vi "Send_Ack_Nack.vi"(8 "Postition to Be Set in":i32[](array[numeric]), 9 "VISA resource name":refnum<visa-resource-name>) -> (2 "Output":enum16{"Error", "NACK", "ACK", "First Send"}(ring), 3 "VISA Out":refnum<visa-resource-name>)   [LabVIEW 2017]
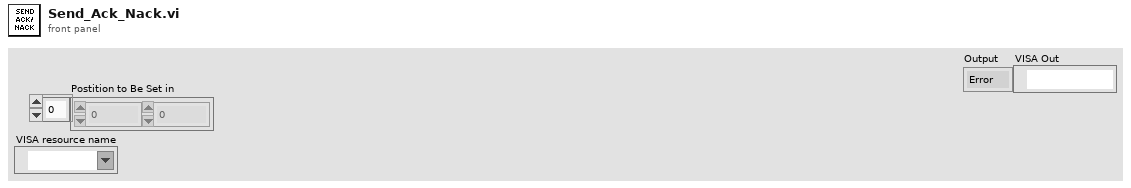
[diagram p1: front panel]
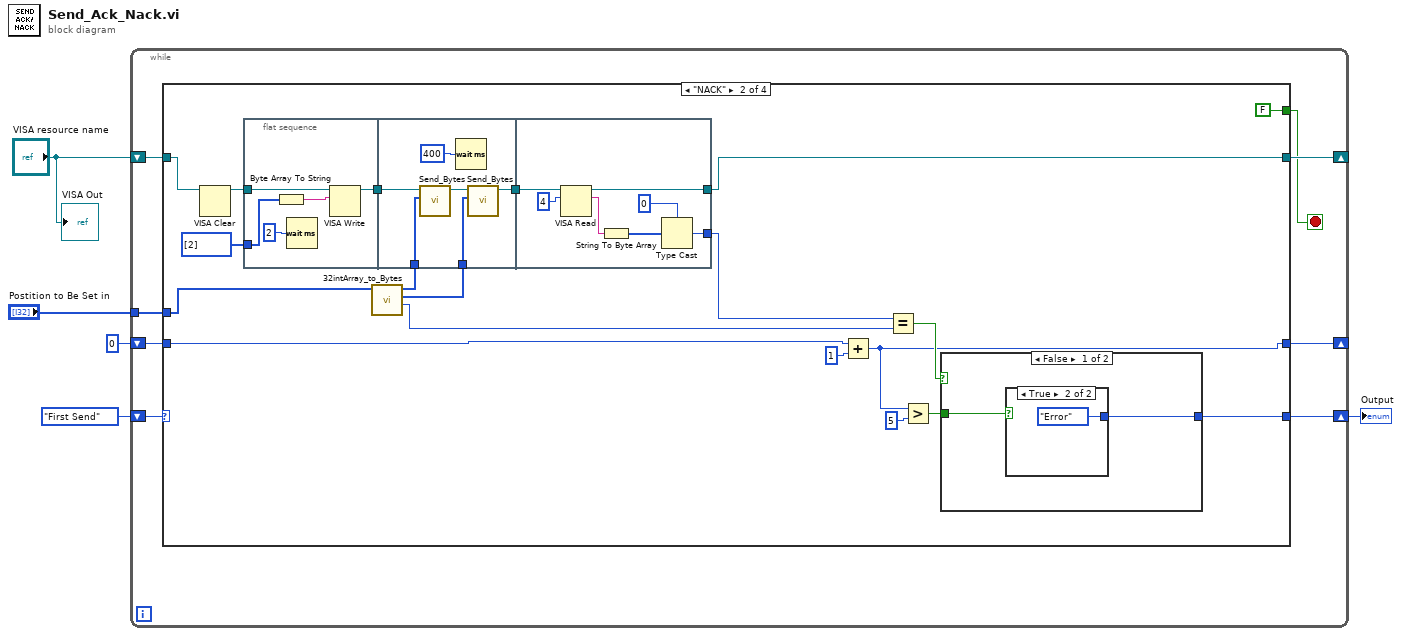
[diagram p0: block diagram]
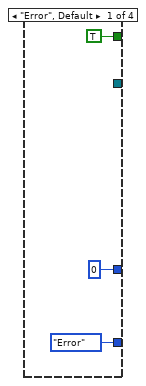
[diagram p2: hidden frame]
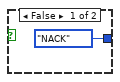
[diagram p3: hidden frame]
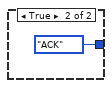
[diagram p4: hidden frame]
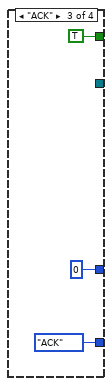
[diagram p5: hidden frame]
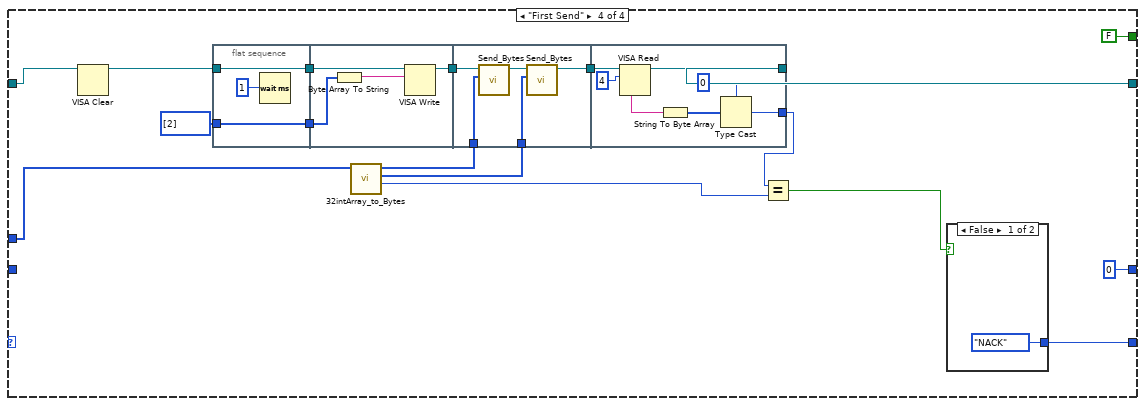
[diagram p6: hidden frame]
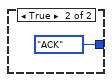
[diagram p7: hidden frame]
diagram:
  n1 = while {
    shift-right: [w9] -> w1
    shift-left: enum16{"Error", "NACK", "ACK", "First Send"}."First Send" -> [w13]
    tunnel: "Postition to Be Set in" -> [w12]
    shift-right: [w6] -> _
    shift-left: 0 -> [w7]
    shift-right: [w11] -> _
    shift-left: "VISA resource name" -> [w10]
    stop <- w8 stop-if-true
    n2 = case shown="\"NACK\"" w13 {
      tunnel: w12 -> [_ w25 _ w73]
      tunnel: [_ w24 _ w70] -> w11
      tunnel: w10 -> [_ w26 _ w63]
      tunnel: [enum16{"Error", "NACK", "ACK", "First Send"}."Error" w23 enum16{"Error", "NACK", "ACK", "First Send"}."ACK" w68] -> w9
      tunnel: [TRUE FALSE TRUE FALSE] -> w8
      tunnel: w7 -> [_ w22 _ _]
      tunnel: [0 w18 0 0] -> w6
      frame "Error", Default {
      }
      frame "NACK" {
        n3 = VISA Clear(VISA resource name=w26) -> (VISA resource name out=w27:refnum<visa-resource-name>)  [unwired: 1 in, 1 out]
        n4 = flat-sequence {
          tunnel: [w45] -> w35
          tunnel: w27 -> [w44]
          tunnel: u8[] [2] -> [w43]
          tunnel: w35 -> [w46]
          tunnel: w29 -> [w48]
          tunnel: [w49] -> w34
          tunnel: w28 -> [w51]
          tunnel: [w57] -> w24
          tunnel: w34 -> [w58]
          tunnel: [w52] -> w32
          frame #0 {
            n5 = Byte Array To String(unsigned byte array=w43) -> (string=w42:string)
            n6 = Wait (ms)(milliseconds to wait=u32 2) -> ()  [unwired: 1 out]
            n7 = VISA Write(VISA resource name=w44, write buffer=w42) -> (VISA resource name out=w45:refnum<visa-resource-name>)  [unwired: 1 in, 2 out]
          }
          frame #1 {
            n8 = call "Send_Bytes.vi"("Array1"=w51, "VISA resource name"=w46) -> ("VISA resource"=w50:refnum<visa-resource-name>)  [unwired: 9 in]
            n9 = Wait (ms)(milliseconds to wait=u32 400) -> ()  [unwired: 1 out]
            n10 = call "Send_Bytes.vi"("Array1"=w48, "VISA resource name"=w50) -> ("VISA resource"=w49:refnum<visa-resource-name>)  [unwired: 9 in]
          }
          frame #2 {
            n11 = VISA Read(VISA resource name=w58, byte count=u32 4) -> (VISA resource name out=w57:refnum<visa-resource-name>, read buffer=w56:string)  [unwired: 1 in, 2 out]
            n12 = String To Byte Array(string=w56) -> (unsigned byte array=w55:u8[])
            n13 = Type Cast(type=0, x=w55) -> (*(type *) &x=w52:i32)
          }
        }
        n14 = call "32intArray_to_Bytes.vi"("Postition to Be Set"=w25) -> ("result"=w31:i32, "Array2"=w29:u8[], "Array1"=w28:u8[])  [unwired: 8 in]
        n15 = Add(x=w22, y=1) -> (x+y=w18:i32)
        n16 = Equal?(x=w32, y=w31) -> (x = y?=w33:bool)
        n17 = Greater?(x=w18, y=5) -> (0:w19:bool)
        n18 = case shown="False" w33 {
          tunnel: [w37 enum16{"Error", "NACK", "ACK", "First Send"}."ACK"] -> w23
          tunnel: w19 -> [w36 _]
          frame False {
            n19 = case shown="True" w36 {
              tunnel: [enum16{"Error", "NACK", "ACK", "First Send"}."NACK" enum16{"Error", "NACK", "ACK", "First Send"}."Error"] -> w37
              frame False {
              }
              frame True {
              }
            }
          }
          frame True {
          }
        }
      }
      frame "ACK" {
      }
      frame "First Send" {
        n20 = VISA Clear(VISA resource name=w63) -> (VISA resource name out=w62:refnum<visa-resource-name>)  [unwired: 1 in, 1 out]
        n21 = flat-sequence {
          tunnel: u8[] [2] -> [w82]
          tunnel: w62 -> [w83]
          tunnel: [w83] -> w65
          tunnel: [w82] -> w64
          tunnel: [w87] -> w78
          tunnel: w65 -> [w86]
          tunnel: w64 -> [w85]
          tunnel: w78 -> [w88]
          tunnel: w75 -> [w89]
          tunnel: [w90] -> w77
          tunnel: w76 -> [w92]
          tunnel: [w98] -> w70
          tunnel: w77 -> [w99]
          tunnel: [w93] -> w71
          frame #0 {
            n22 = Wait (ms)(milliseconds to wait=u32 1) -> ()  [unwired: 1 out]
          }
          frame #1 {
            n23 = Byte Array To String(unsigned byte array=w85) -> (string=w84:string)
            n24 = VISA Write(VISA resource name=w86, write buffer=w84) -> (VISA resource name out=w87:refnum<visa-resource-name>)  [unwired: 1 in, 2 out]
          }
          frame #2 {
            n25 = call "Send_Bytes.vi"("Array1"=w92, "VISA resource name"=w88) -> ("VISA resource"=w91:refnum<visa-resource-name>)  [unwired: 9 in]
            n26 = call "Send_Bytes.vi"("Array1"=w89, "VISA resource name"=w91) -> ("VISA resource"=w90:refnum<visa-resource-name>)  [unwired: 9 in]
          }
          frame #3 {
            n27 = VISA Read(VISA resource name=w99, byte count=u32 4) -> (VISA resource name out=w98:refnum<visa-resource-name>, read buffer=w97:string)  [unwired: 1 in, 2 out]
            n28 = String To Byte Array(string=w97) -> (unsigned byte array=w96:u8[])
            n29 = Type Cast(type=0, x=w96) -> (*(type *) &x=w93:i32)
          }
        }
        n30 = call "32intArray_to_Bytes.vi"("Postition to Be Set"=w73) -> ("result"=w72:i32, "Array2"=w75:u8[], "Array1"=w76:u8[])  [unwired: 8 in]
        n31 = Equal?(x=w71, y=w72) -> (x = y?=w69:bool)
        n32 = case shown="False" w69 {
          tunnel: [enum16{"Error", "NACK", "ACK", "First Send"}."NACK" enum16{"Error", "NACK", "ACK", "First Send"}."ACK"] -> w68
          frame False {
          }
          frame True {
          }
        }
      }
    }
  }
  "Output" <- w1
  "VISA Out" <- "VISA resource name"
